vi "Page Explorer.vi"   [LabVIEW 2020]
types:
  T1 = enum32{"Invalid", "Standard", "Closed", "Hidden", "Minimized", "Maximized"}
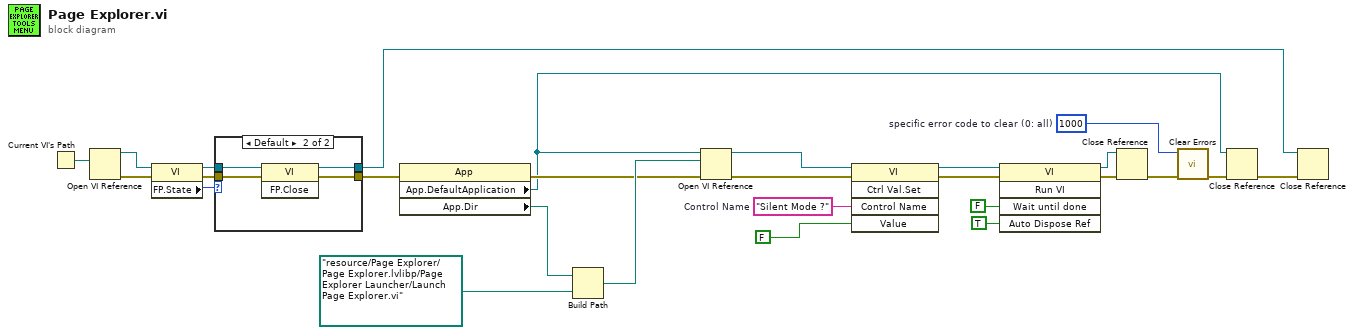
[diagram p0: block diagram]
diagram:
  w15 = 1000  # specific error code to clear (0: all)
  w19 = "Silent Mode ?"  # Control Name
  n1 = Current VI's Path() -> (path=w14:path)
  n2 = Open VI Reference(vi path=w14) -> (vi reference=w11:refnum<vi>, error out=w10:errorcluster)  [unwired: 5 in]
  n3 = property class="VI"(reference=w11, error in=w10) -> (reference out=w12:refnum<vi>, error out=w13:errorcluster, "FP.State"=w9:T1)
  n4 = case shown="Default" w9 {
    tunnel: [w29 w33] -> w8
    tunnel: w13 -> [w29 w32]
    tunnel: w12 -> [w28 w31]
    tunnel: [w28 w30] -> w7
    frame "Invalid", "Closed" {
    }
    frame Default {
      n5 = invoke class="VI" method="FP.Close"(reference=w31, error in=w32) -> (reference out=w30:refnum<vi>, error out=w33:errorcluster)  [unwired: 1 in, 1 out]
    }
  }
  n6 = property class="App"(error in=w8) -> (error out=w24:errorcluster, "App.DefaultApplication"=w1:refnum<vi>, "App.Dir"=w27:path)  [unwired: 1 in, 1 out]
  n7 = Build Path(base path=w27, name or relative path=path "resource/Page Explorer/Page Explorer.lvlibp/Page Explorer Launcher/Launch Page Explorer.vi" ("vi path")) -> (appended path=w25:path)
  n8 = Open VI Reference(application reference (local)=w1, vi path=w25, error in (no error)=w24) -> (vi reference=w17:refnum<vi>, error out=w16:errorcluster)  [unwired: 3 in]
  n9 = invoke class="VI" method="Ctrl Val.Set"(reference=w17, error in=w16, "Control Name"=w19, "Value"=FALSE ("Auto Dispose Reference")) -> (reference out=w20:refnum<vi>, error out=w21:errorcluster)  [unwired: 1 in, 3 out]
  n10 = invoke class="VI" method="Run VI"(reference=w20, error in=w21, "Wait until done"=FALSE ("Wait Until Done"), "Auto Dispose Ref"=TRUE ("Auto Dispose Reference")) -> (reference out=w5:refnum<vi>, error out=w6:errorcluster)  [unwired: 1 in, 3 out]
  n11 = Close Reference(reference=w5, error in (no error)=w6) -> (error out=w3:errorcluster)
  n12 = call <vilib>:"Clear Errors.vi"("error in (no error)"=w3, "specific error code to clear (0: all)"=w15) -> ("error out"=w4:errorcluster)  [unwired: 4 in, 1 out]
  n13 = Close Reference(reference=w1, error in (no error)=w4) -> (error out=w2:errorcluster)
  n14 = Close Reference(reference=w7, error in (no error)=w2) -> ()  [unwired: 1 out]
